vi "AMC Destroy Message Queue.vi"(8 "error in (no error)":errorcluster, 11 "Message Queue in":T1) -> (0 "error out":errorcluster, 3 "Queue Name":string)   [LabVIEW 2017]
doc: "Release the reference to the event queue and return any remaing events."
uses:
  subVIs/TypeDefs/amc_Message Queue.ctl
  subVIs/TypeDefs/amc_Message.ctl
  Tools/Keyed Array/Tools_KeyedArray KeyedArray.ctl
  Queue Registry/TypeDefs/amc_QueueRegistryMethod.ctl
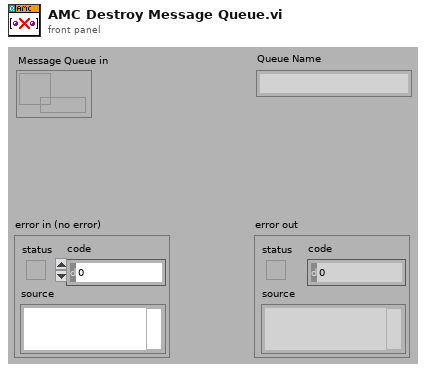
[diagram p1: front panel]
types:
  T1 = typedef "amc_Message Queue.ctl" = refnum<queue>
  T2 = typedef "amc_QueueRegistryMethod.ctl" = enum16{"Initialize", "Add Queue", "Set Properties", "Get Queue by Index", "Get Queue by Name", "Remove Queue", "Remove All Queues"}
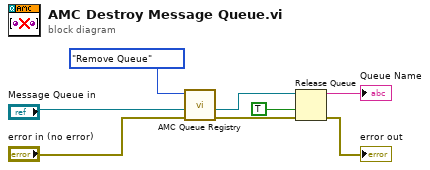
[diagram p0: block diagram]
diagram:
  n1 = call "AMC Queue Registry.vi"("error in (no error)"="error in (no error)", "Message Queue in"="Message Queue in", "Method"=amc_QueueRegistryMethod."Remove Queue") -> ("error out"=w2:errorcluster, "Message Queue out"=w1:T1)  [unwired: 2 in, 5 out]
  n2 = Release Queue(queue=w1, force destroy? (F)=TRUE, error in (no error)=w2) -> (queue name=→"Queue Name":string, error out=→"error out":errorcluster)  [unwired: 1 out]
